vi "addNode.vi"(8 "error in (no error)":errorcluster, 9 "superNode Path":string, 10 "Data Class":string, 11 "xceRootNode in":refnum<class "xceRootNode.lvclass">) -> (0 "error out":errorcluster, 3 "xceRootNode out":refnum<class "xceRootNode.lvclass">)   [LabVIEW 2013, in "xceRootNode.lvclass"]
doc: "Adds a node in the tree data structure, and the tree control."
uses:
  xceRootNode.lvclass
  xceDataNode/xceDataNode.lvclass
  xceRootNode.lvclass/xceRootNode.ctl
  xceNode/xceNode.lvclass
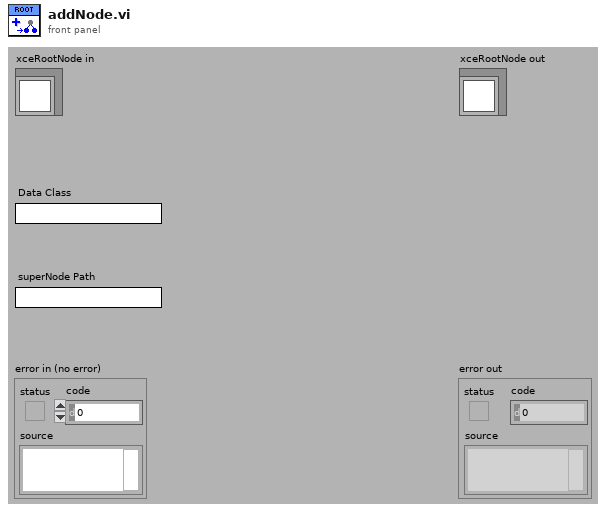
[diagram p1: front panel]
types:
  T1 = cluster{"className":string, "classAlias":string}[]
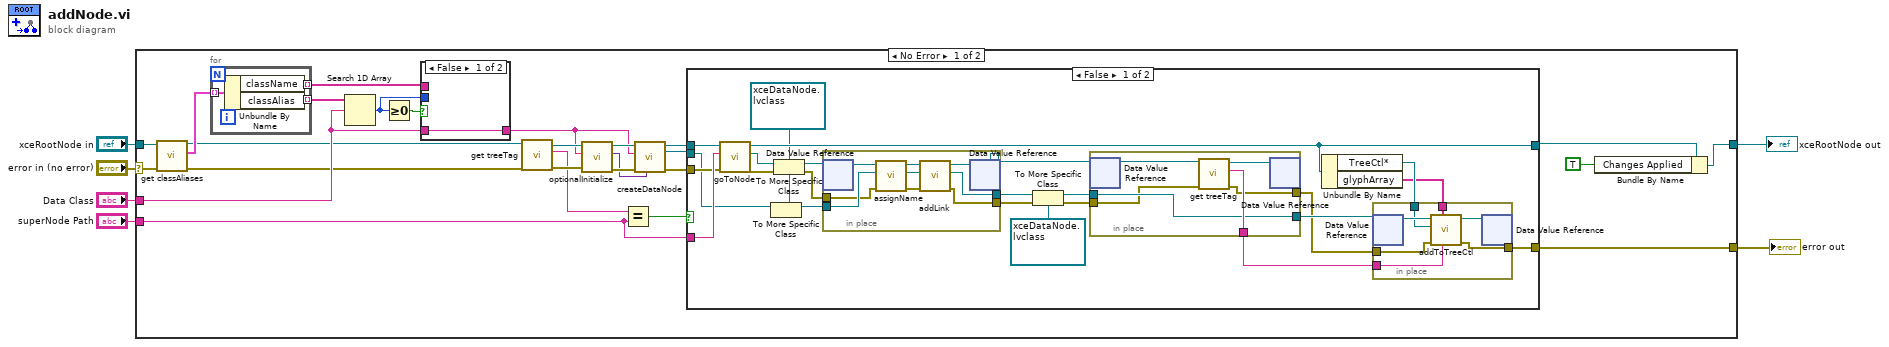
[diagram p0: block diagram]
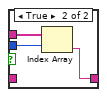
[diagram p2: hidden frame]
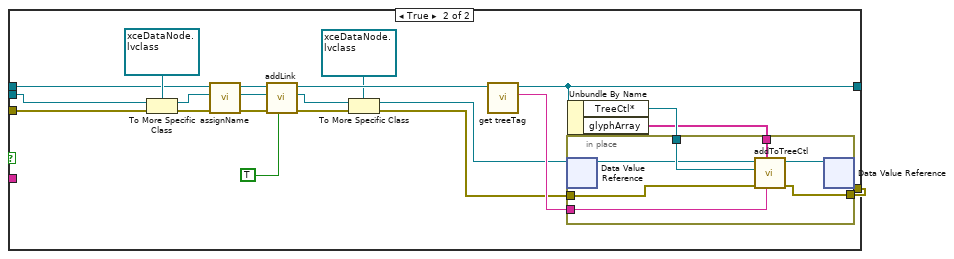
[diagram p3: hidden frame]
diagram:
  n1 = case shown="No Error" "error in (no error)" {
    selector: "error in (no error)" -> [w22 w114]
    tunnel: [w28 w114] -> w5
    tunnel: [w24 w113] -> w3
    tunnel: "xceRootNode in" -> [w23 w113]
    tunnel: "Data Class" -> [w19 _]
    tunnel: "superNode Path" -> [w27 _]
    frame No Error {
      n2 = call "get classAliases.vi"("error in (no error)"=w22, "xceRootNode in"=w23) -> ("error out"=w15:errorcluster, "classAliases"=w21:T1, "xceRootNode out"=w16:refnum<class "xceRootNode.lvclass">)  [unwired: 7 in]
      n3 = for {
        tunnel: w21 -> [w39] mode=indexing
        tunnel: [w38] -> w14 mode=indexing
        tunnel: [w37] -> w18 mode=indexing
        n4 = Unbundle By Name(w39) -> ("className"=w38:string, "classAlias"=w37:string)
      }
      n5 = Search 1D Array(1D array=w18, element=w19) -> (index of element=w17:i32)  [unwired: 1 in]
      n6 = Greater Or Equal To 0?(x=w17) -> (x >= 0?=w20:bool)
      n7 = case shown="False" w20 {
        tunnel: w19 -> [w33 _]
        tunnel: w14 -> [_ w36]
        tunnel: w17 -> [_ w35]
        tunnel: [w33 w34] -> w7
        frame False {
        }
        frame True {
          n8 = Index Array(array=w36, index=w35) -> (element=w34:string)
        }
      }
      n9 = call "get treeTag.vi"("error in (no error)"=w15, "xceNode in"=w16) -> ("error out"=w12:errorcluster, "treeTag"=w8:string, "xceNode out"=w13:refnum<class "xceRootNode.lvclass">)  [unwired: 7 in]
      n10 = call-dynamic "optionalInitialize.vi"("error in (no error)"=w12, "Class Name"=w7, "xceRootNode in"=w13) -> ("error out"=w10:errorcluster, "optional Data"=w9:variant, "xceRootNode out"=w11:refnum<class "xceRootNode.lvclass">)  [unwired: 6 in]
      n11 = Equal?(x=w8, y=w27) -> (x = y?=w32:bool)
      n12 = call "createDataNode.vi"("optional"=w9, "error in (no error)"=w10, "Data Class"=w7, "xceRootNode in"=w11) -> ("error out"=w29:errorcluster, "newNode*"=w31:refnum<data-value>, "xceRootNode out"=w30:refnum<class "xceRootNode.lvclass">)  [unwired: 5 in]
      n13 = case shown="False" w32 {
        tunnel: w30 -> [w62 w97]
        tunnel: w29 -> [w60 w96]
        tunnel: w31 -> [w44 w98]
        tunnel: [w56 w103] -> w26
        tunnel: [w51 w101] -> w28
        tunnel: w27 -> [w61 _]
        frame False {
          w43 = refnum<data-value> refnum ("data value reference")
          n14 = call "goToNode.vi"("error in (no error)"=w60, "Node Path"=w61, "xceNode in"=w62) -> ("error out"=w47:errorcluster, "goToNode* out"=w49:refnum<data-value>, "xceNode out"=w56:refnum<class "xceRootNode.lvclass">)  [unwired: 6 in]
          n15 = To More Specific Class(target class=w43, reference=w44) -> (specific class reference=w45:refnum<data-value>)  [unwired: 1 in, 1 out]
          n16 = To More Specific Class(target class=w43, reference=w49, error in=w47) -> (specific class reference=w48:refnum<data-value>, error out=w46:errorcluster)
          n17 = in-place {
            in-place-border: w45 -> [w66]
            in-place-border: [w70] -> w50
            in-place-border: w46 -> [w63]
            in-place-border: [w69] -> w42
            n18 = in-place-dvr #1(w48) -> (w67:refnum<class "xceDataNode.lvclass">)  [unwired: 1 out]
            n19 = call "assignName.vi"("error in (no error)"=w63, "subNode in"=w66, "superNode in"=w67) -> ("error out"=w64:errorcluster, "subNode out"=w65:refnum<data-value>, "superNode out"=w68:refnum<class "xceDataNode.lvclass">)  [unwired: 6 in]
            n20 = call "addLink.vi"("error in (no error)"=w64, "subNode in"=w65, "superNode in"=w68) -> ("error out"=w69:errorcluster, "subNode out"=w70:refnum<data-value>, "superNode out"=w71:refnum<class "xceDataNode.lvclass">)  [unwired: 6 in]
            n21 = in-place-dvr #1(w71) -> (w41:refnum<data-value>)  [unwired: 1 out]
          }
          n22 = To More Specific Class(target class=refnum<data-value> refnum ("data value reference"), reference=w50, error in=w42) -> (specific class reference=w58:refnum<data-value>, error out=w57:errorcluster)
          n23 = in-place {
            in-place-border: w58 -> [w80]
            in-place-border: w57 -> [w79]
            in-place-border: [w80] -> w55
            in-place-border: [w84] -> w52
            in-place-border: [w82] -> w53
            n24 = in-place-dvr #2(w41) -> (w81:refnum<class "xceDataNode.lvclass">)  [unwired: 1 out]
            n25 = call "get treeTag.vi"("error in (no error)"=w79, "xceNode in"=w81) -> ("error out"=w82:errorcluster, "treeTag"=w84:string, "xceNode out"=w83:refnum<class "xceDataNode.lvclass">)  [unwired: 7 in]
            n26 = in-place-dvr #2(w83) -> ()  [unwired: 2 out]
          }
          n27 = Unbundle By Name(w56) -> ("TreeCtl*"=w54:refnum<vi>, "glyphArray"=w40:string[])
          n28 = in-place {
            in-place-border: w54 -> [w76]
            in-place-border: w53 -> [w75]
            in-place-border: w52 -> [w74]
            in-place-border: [w73] -> w51
            in-place-border: w40 -> [w72]
            n29 = in-place-dvr #3(w55) -> (w78:refnum<class "xceDataNode.lvclass">)  [unwired: 1 out]
            n30 = call "addToTreeCtl.vi"("ParentTreeTag"=w74, "glyphArray"=w72, "error in (no error)"=w75, "TreeCtl*"=w76, "xceDataNode in"=w78) -> ("error out"=w73:errorcluster, "xceDataNode out"=w77:refnum<class "xceDataNode.lvclass">)  [unwired: 5 in]
            n31 = in-place-dvr #3(w77) -> ()  [unwired: 2 out]
          }
        }
        frame True {
          n32 = To More Specific Class(target class=refnum<data-value> refnum ("data value reference"), reference=w98, error in=w96) -> (specific class reference=w100:refnum<data-value>, error out=w99:errorcluster)
          n33 = call "assignName.vi"("error in (no error)"=w99, "subNode in"=w100, "superNode in"=w97) -> ("error out"=w92:errorcluster, "subNode out"=w93:refnum<data-value>, "superNode out"=w95:refnum<class "xceRootNode.lvclass">)  [unwired: 6 in]
          n34 = call "addLink.vi"("Append to End"=TRUE, "error in (no error)"=w92, "subNode in"=w93, "superNode in"=w95) -> ("error out"=w91:errorcluster, "subNode out"=w89:refnum<data-value>, "superNode out"=w94:refnum<class "xceRootNode.lvclass">)  [unwired: 5 in]
          n35 = To More Specific Class(target class=refnum<data-value> refnum ("data value reference"), reference=w89, error in=w91) -> (specific class reference=w88:refnum<data-value>, error out=w90:errorcluster)
          n36 = call "get treeTag.vi"("xceNode in"=w94) -> ("treeTag"=w102:string, "xceNode out"=w103:refnum<class "xceRootNode.lvclass">)  [unwired: 8 in, 1 out]
          n37 = Unbundle By Name(w103) -> ("TreeCtl*"=w104:refnum<vi>, "glyphArray"=w86:string[])
          n38 = in-place {
            in-place-border: w104 -> [w111]
            in-place-border: w90 -> [w110]
            in-place-border: [w109] -> w101
            in-place-border: w102 -> [w107]
            in-place-border: w86 -> [w106]
            n39 = in-place-dvr #4(w88) -> (w108:refnum<class "xceDataNode.lvclass">)  [unwired: 1 out]
            n40 = call "addToTreeCtl.vi"("ParentTreeTag"=w107, "glyphArray"=w106, "error in (no error)"=w110, "TreeCtl*"=w111, "xceDataNode in"=w108) -> ("error out"=w109:errorcluster, "xceDataNode out"=w112:refnum<class "xceDataNode.lvclass">)  [unwired: 5 in]
            n41 = in-place-dvr #4(w112) -> ()  [unwired: 2 out]
          }
        }
      }
      n42 = Bundle By Name(cluster=w26, "Changes Applied"=TRUE) -> (w24:refnum<class "xceRootNode.lvclass">)
    }
    frame Error {
    }
  }
  "error out" <- w5
  "xceRootNode out" <- w3
